vi "Insert BD Enum.vi"(8 "error in (no error)":errorcluster, 9 "path":path, 10 "BD Location":T1, 11 "Owner  in":refnum<vi>) -> (0 "error out":errorcluster, 2 "Enum out":refnum<vi>, 3 "Owner  out":refnum<vi>)   [LabVIEW 2019, in "gRPC Scripting Tools.lvlib"]
uses:
  gRPC Scripting Tools.lvlib
  <vilib>/Utility/miscctls.llb/LVPointTypeDef.ctl
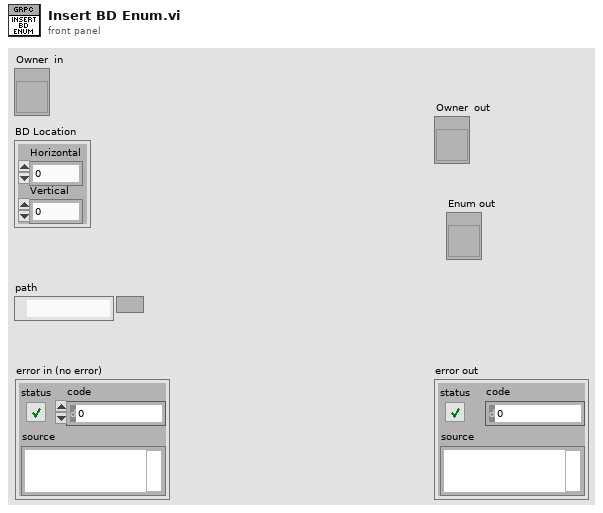
[diagram p1: front panel]
types:
  T1 = typedef "LVPointTypeDef.ctl" = cluster{"Horizontal":i16, "Vertical":i16}
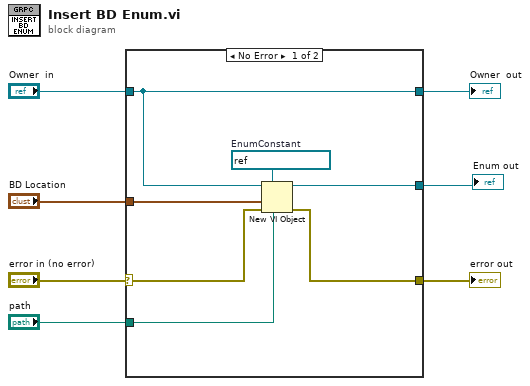
[diagram p0: block diagram]
diagram:
  n1 = case shown="No Error" "error in (no error)" {
    selector: "error in (no error)" -> [w8 w16]
    tunnel: "Owner  in" -> [w9 w15]
    tunnel: "path" -> [w14 _]
    tunnel: "BD Location" -> [w13 _]
    tunnel: [w12 w16] -> w4
    tunnel: [w10 _] -> w3
    tunnel: [w9 w15] -> w2
    frame No Error {
      w11 = refnum<vi> refnum  # EnumConstant
      n2 = New VI Object(vi object class=w11, owner refnum=w9, position/next to=w13, 6:w14, 8:w8) -> (object refnum=w10:refnum<vi>, 0:w12:errorcluster)  [unwired: 1 in, 2 out]
    }
    frame Error {
    }
  }
  "error out" <- w4
  "Owner  out" <- w2
  "Enum out" <- w3
